vi "AbsolutePlungerPositionStatus (SubVI).vi"(11 "VISA Refnum in":refnum<visa-resource-name>) -> (3 "read buffer":string)   [LabVIEW 2020]
uses:
  <vilib>/Instr/_visa.llb/VISA Configure Serial Port (Instr).vi
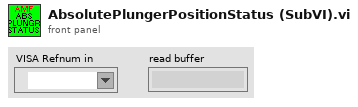
[diagram p1: front panel]
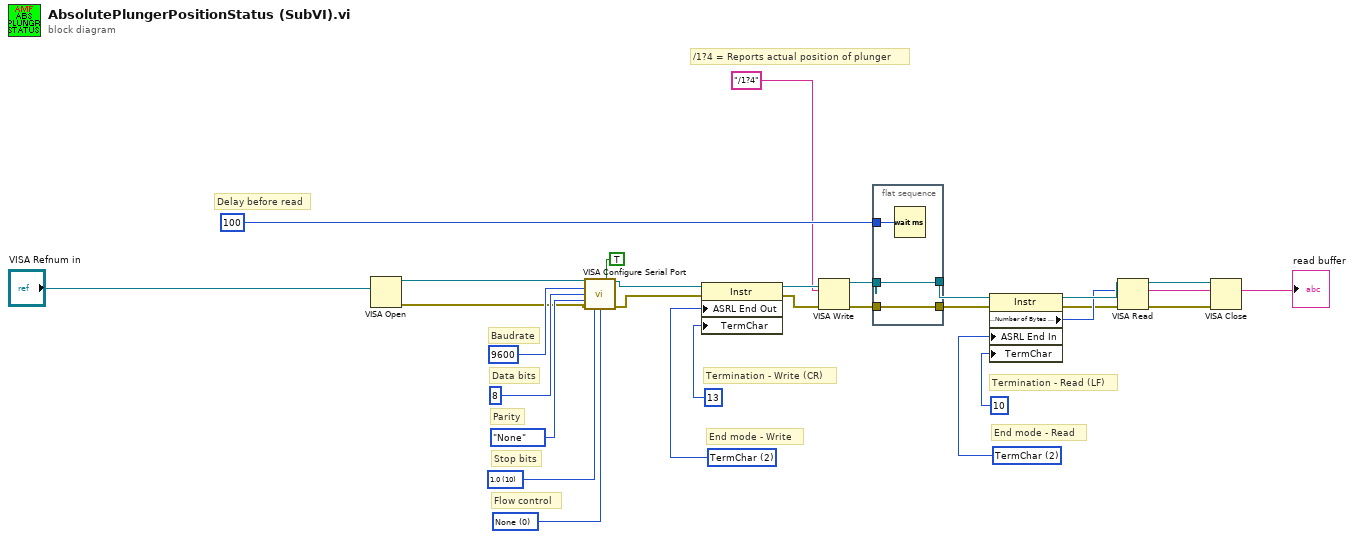
[diagram p0: block diagram]
diagram:
  w28 = u16 2 items=["None", "Last Bit", "TermChar"] ("Serial Settings:End Mode for Reads")
  w25 = u16 2 items=["None", "Last Bit", "TermChar", "Break"] ("Serial Settings:End Mode for Writes")
  w24 = u16 0 items=["None", "XON/XOFF", "RTS/CTS", "XON/XOFF & RTS/CTS", "DTR/DSR", "XON/XOFF & DTR/DSR"] ("flow control (0:none)")
  w23 = u16 10 items=["1.0"=10, "1.5"=15, "2.0"=20] ("stop bits (10: 1 bit)")
  # "/1?4 = Reports actual position of plunger"
  # "End mode - Read"
  # "Termination - Read (LF)"
  # "End mode - Write"
  # "Termination - Write (CR)"
  # "Flow control"
  # "Stop bits"
  # "Parity"
  # "Data bits"
  # "Baudrate"
  # "Delay before read"
  n1 = VISA Open(VISA resource name="VISA Refnum in") -> (VISA resource name=w15:refnum<visa-resource-name>, error out=w16:errorcluster)  [unwired: 4 in]
  n2 = call-poly "VISA Configure Serial Port"("VISA resource name"=w15, "Enable Termination\nChar (T)"=TRUE, "baud rate (9600)"=u32 9600, "data bits (8)"=u16 8, "parity (0:none)"=enum16{"None", "Odd", "Even", "Mark", "Space"}."None", "error in (no error)"=w16, "stop bits (10: 1 bit)"=w23, "flow control (0:none)"=w24) -> ("VISA resource name out"=w8:refnum<visa-resource-name>, "error out"=w9:errorcluster)  [unwired: 1 in, 5 out]
  n3 = property class="Instr"(reference=w8, error in=w9, "ASRL End Out"=w25, "TermChar"=u8 13 ("Message Based Settings:Termination Character")) -> (reference out=w10:refnum<visa-resource-name>, error out=w11:errorcluster)
  n4 = VISA Write(VISA resource name=w10, write buffer="/1?4", error in (no error)=w11) -> (VISA resource name out=w4:refnum<visa-resource-name>, error out=w2:errorcluster)  [unwired: 1 out]
  n5 = flat-sequence {
    tunnel: w2 -> [w31]
    tunnel: [w31] -> w3
    tunnel: w4 -> [w30]
    tunnel: [w30] -> w19
    tunnel: u32 100 ("delay before read (ms)") -> [w32]
    frame #0 {
      n6 = Wait (ms)(milliseconds to wait=w32) -> ()  [unwired: 1 out]
    }
  }
  n7 = property class="Instr"(reference=w19, error in=w3, "ASRL End In"=w28, "TermChar"=u8 10 ("Message Based Settings:Termination Character")) -> (reference out=w18:refnum<visa-resource-name>, error out=w6:errorcluster, "Serial Settings:Number of Bytes at Serial Port"=w7:u32)
  n8 = VISA Read(VISA resource name=w18, byte count=w7, error in (no error)=w6) -> (VISA resource name out=w13:refnum<visa-resource-name>, read buffer=→"read buffer":string, error out=w14:errorcluster)  [unwired: 1 out]
  n9 = VISA Close(VISA resource name=w13, error in (no error)=w14) -> ()  [unwired: 1 out]
